vi "Update W.vi"(8 "error in (no error)":errorcluster, 10 "SLAM In":T3, 11 "New LM's In":T2(array[cluster])) -> (0 "error out":errorcluster, 2 "SLAM Out":T3, 3 "New LM's Out":T2(array[cluster]))   [LabVIEW 2009]
uses:
  <vilib>/Analysis/Matrix/Datatypes/RealMatrix.ctl
  Controls/SLAM.ctl
  <vilib>/Analysis/Matrix/NI_Matrix.lvlib
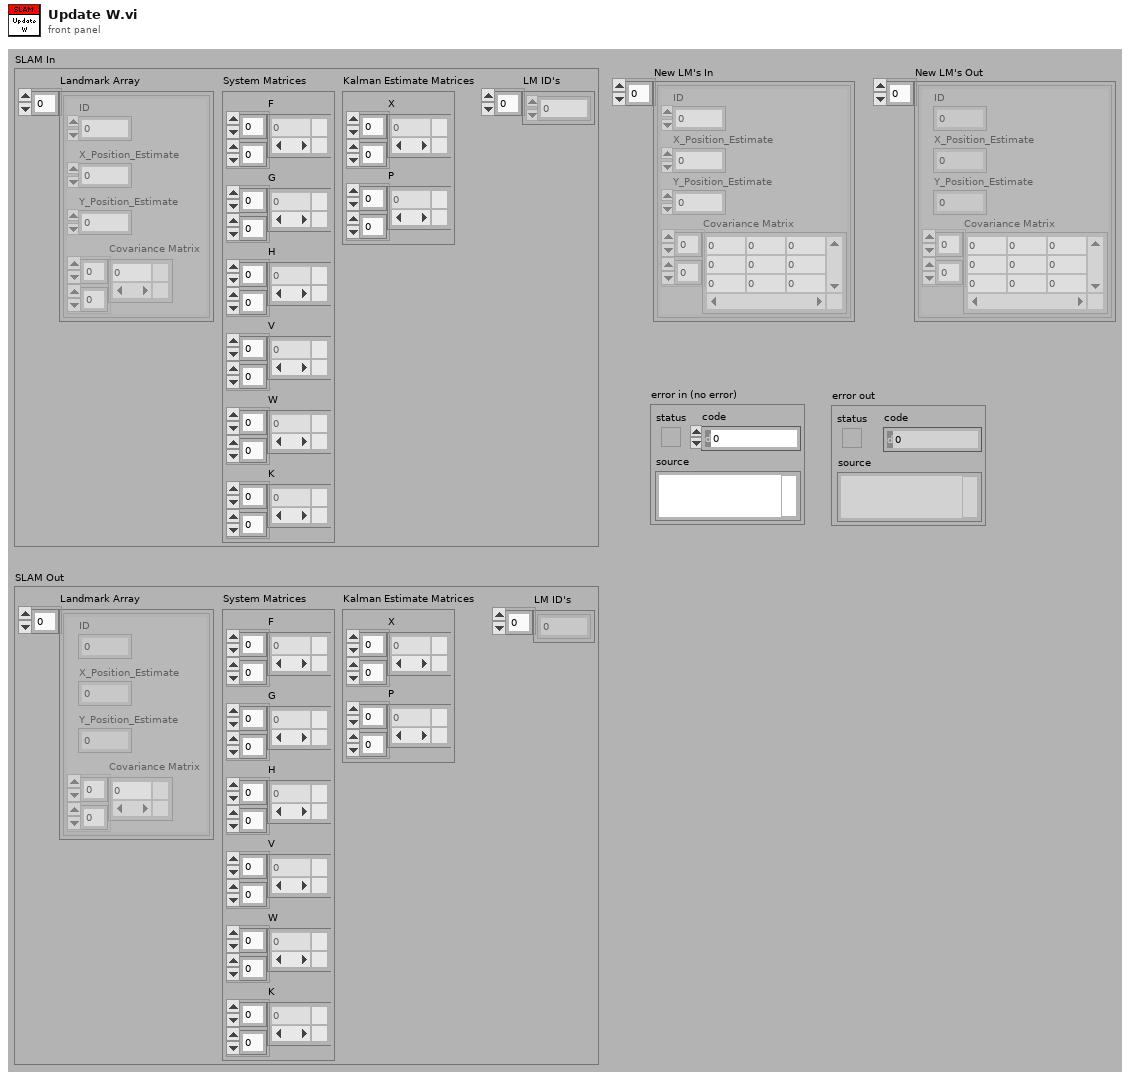
[diagram p1: front panel]
types:
  T1 = typedef "NI_Matrix.lvlib/RealMatrix.ctl" = dbl[][]
  T2 = cluster{"ID":dbl, "X_Position_Estimate":dbl, "Y_Position_Estimate":dbl, "Covariance Matrix":T1}[]
  T3 = typedef "SLAM.ctl" = cluster{"Landmark Array":cluster{"ID":dbl, "X_Position_Estimate":dbl, "Y_Position_Estimate":dbl, "Covariance Matrix":T1}[], "System Matrices":cluster{"F":T1, "G":T1, "H":T1, "V":T1, "W":T1, "K":T1}, "Kalman Estimate Matrices":cluster{"X":T1, "P":T1}, "LM ID's":dbl[]}
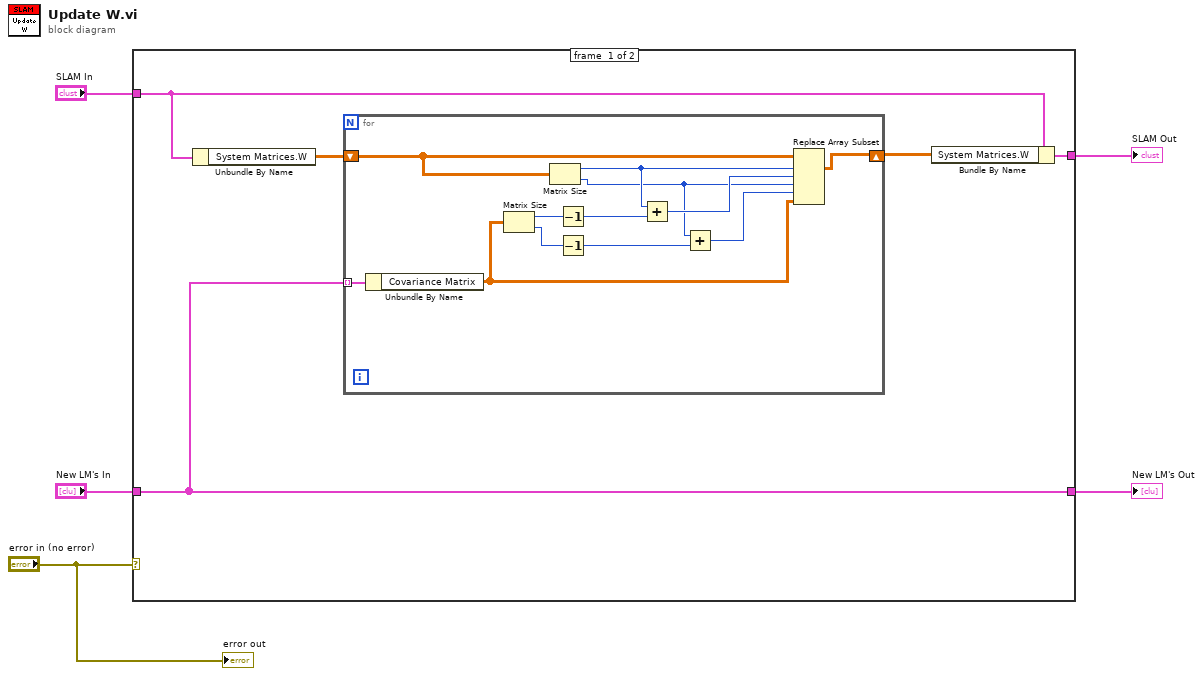
[diagram p0: block diagram]
diagram:
  n1 = case shown="No Error" "error in (no error)" {
    tunnel: "SLAM In" -> [w10 w23]
    tunnel: "New LM's In" -> [w6 w24]
    tunnel: [w9 w23] -> w3
    tunnel: [w6 w24] -> w2
    frame #0 {
      n2 = Unbundle By Name(w10) -> ("System Matrices.W"=w7:T1)
      n3 = for {
        shift-right: [w17] -> w8
        shift-left: w7 -> [w16]
        tunnel: w6 -> [w15] mode=indexing
        n4 = Unbundle By Name(w15) -> ("Covariance Matrix"=w11:T1)
        n5 = Matrix Size(0:w11) -> (1:w14:i32, 2:w13:i32)
        n6 = Matrix Size(0:w16) -> (1:w22:i32, 2:w20:i32)
        n7 = Decrement(x=w14) -> (x-1=w18:i32)
        n8 = Decrement(x=w13) -> (x-1=w12:i32)
        n9 = Add(x=w22, y=w18) -> (x+y=w21:i32)
        n10 = Add(x=w20, y=w12) -> (x+y=w19:i32)
        n11 = Replace Array Subset(array=w16, new element=w11, index (dim 0)=w22, index (dim 1)=w21, index (dim 2)=w20, index (dim 3)=w19) -> (w17:T1)
      }
      n12 = Bundle By Name(cluster=w10, "System Matrices.W"=w8) -> (w9:T3)
    }
    frame #1 {
    }
  }
  "New LM's Out" <- w2
  "SLAM Out" <- w3
  "error out" <- "error in (no error)"
